vi "468_SignalRead_OutputOnce_2026.vi"() -> ()   [LabVIEW 2025]
panel:
  out "error out":errorcluster
  out "Signal plot":dbl(graph)
  in  "Filename":path=path "G:/498F-599G/Lab03/426_signal_104-I_125Hz.lvm"
  in  "millisecond multiple":u32=8
  in  "stop":bool
  out "Filename Out":path
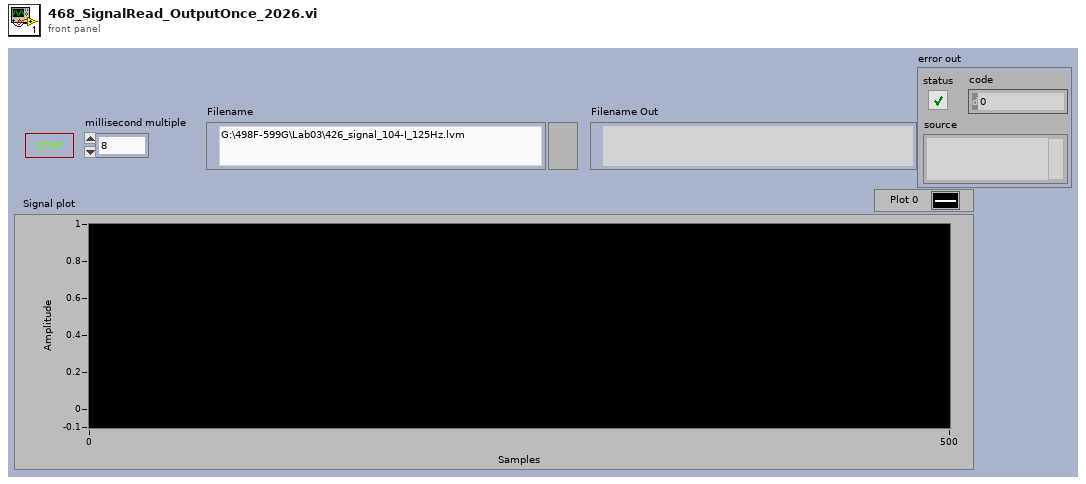
[diagram p1: front panel]
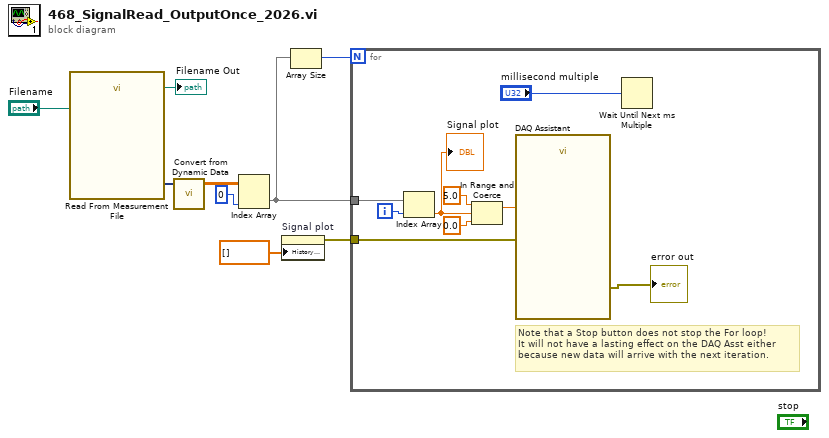
[diagram p0: block diagram]
diagram:
  n1 = call "Read From Measurement File"("Filename"="Filename") -> ("Filename Out"=→"Filename Out":path, "Signals"=w5:dynamicdata)  [unwired: 5 in, 4 out]
  n2 = call "Convert from Dynamic Data"("Dynamic Data Type"=w5) -> ("Array"=w4:dbl[][])  [unwired: 3 in]
  n3 = Index Array(array=w4, index (col)=0 ("disabled index (col)")) -> (element=w3:dbl[])  [unwired: 1 in]
  n4 = property on="Signal plot" class="WFChart (strict)"("History Data"=dbl[] []) -> (error out=w1:errorcluster)  [unwired: 2 in, 1 out]
  n5 = Array Size(array=w3) -> (size(s)=w7:i32)
  n6 = for {
    N: w7 -> [_]
    tunnel: w3 -> [w13]
    tunnel: w1 -> [w11]
    i -> [w14]
    # "Note that a Stop button does not stop the For loop!\nIt will not have a lasting effect on the DAQ Asst either\nbecause new data will arrive with the next iteration."
    n7 = Index Array(array=w13, index=w14) -> (element=w15:dbl)
    "Signal plot" <- w15
    n8 = In Range and Coerce(upper limit=sgl 5.0, x=w15, lower limit=sgl 0.0) -> (coerced(x)=w12:dbl)  [unwired: 1 out]
    n9 = call "DAQ Assistant"("data"=w12, "error in"=w11) -> ("error out"=→"error out":errorcluster)  [unwired: 16 in, 1 out]
    n10 = Wait Until Next ms Multiple(millisecond multiple="millisecond multiple") -> ()  [unwired: 1 out]
  }
